vi "Rec Move To Next Record (R).vi"(8 "error in (no error)":errorcluster, 11 "recordset reference":T1) -> (0 "error out":errorcluster, 3 "recordset reference out":T1)   [LabVIEW 2012, in "NI_Database_API_64.lvlib"]
doc: "Moves the cursor to point to the next record in the recordset identified by the reference. Wire data to the reference input to determine the polymorphic instance to use or manually select the instance."
uses:
  NI_Database_API_64.lvlib
  Rec ObjectReference.ctl
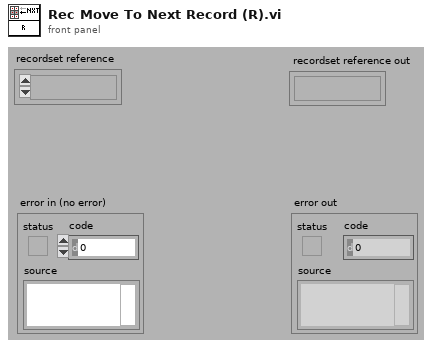
[diagram p1: front panel]
types:
  T1 = typedef "NI_Database_API_64.lvlib/Rec ObjectReference.ctl" = refnum<k1>
  T2 = typedef "NI_Database_API_64.lvlib/Rec DataMembers.ctl" = cluster{"ADODB._Recordset":refnum<k7>, "Connection":T3}
  T3 = typedef "NI_Database_API_64.lvlib/Conn ObjectReference.ctl" = refnum<k1>
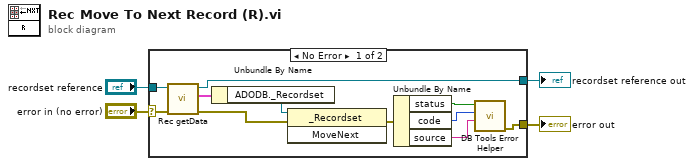
[diagram p0: block diagram]
diagram:
  n1 = case shown="No Error" "error in (no error)" {
    selector: "error in (no error)" -> [w5 w17]
    tunnel: "recordset reference" -> [w15 w16]
    tunnel: [w11 w16] -> w3
    tunnel: [w7 w17] -> w2
    frame No Error {
      n2 = call "Rec getData.vi"("error in (no error)"=w5, "recordset reference"=w15) -> ("error out"=w13:errorcluster, "data"=w14:T2, "recordset reference out"=w11:T1)  [unwired: 3 out]
      n3 = Unbundle By Name(w14) -> ("ADODB._Recordset"=w12:refnum<k7>)
      n4 = invoke class="_Recordset" method="MoveNext"(reference=w12, error in=w13) -> (error out=w8:errorcluster)  [unwired: 1 in, 2 out]
      n5 = Unbundle By Name(w8) -> ("status"=w9:bool, "code"=w6:i32, "source"=w10:string)
      n6 = call "DB Tools Error Helper.vi"("source"=w10, "code"=w6, "status"=w9) -> ("error out"=w7:errorcluster)  [unwired: 1 in, 7 out]
    }
    frame Error {
    }
  }
  "recordset reference out" <- w3
  "error out" <- w2
